vi "Main Window.vi"() -> ()   [LabVIEW 2015]
uses:
  Control Button/Exit.ctl
  Control Button/login.ctl
  Control Button/Logout.ctl
  Control Button/setting.ctl
  Control Button/report.ctl
  Control Button/Manual.ctl
  Control Button/Start.ctl
  Enqueue/Main window Seq/Test selection_1.ctl
  Enqueue/Main window Seq/Test seq_1.ctl
  Galobal variable_TI.vi
  Project Setup/Globle Variable/GR_Servo.vi
panel:
  out "Company Name  2":string
  out "Error":bool
  out "User Name":string
  out "error out":errorcluster
  out "x = y?":bool
  out "Company Name":string
  in  "Sign In":T1
  out "Boolean":bool
  in  "Dashbord":T6
  in  "Login Window":T8 {"User Name" items=["admin", "mmum", "a", "AJAY Kumar", "", "", "", "", "", "", "", "", "", "", "", "", "", "", "", "", "", "", "", "", "", "", "", "", "", "", "", ""]}
  in  "Exit":T9
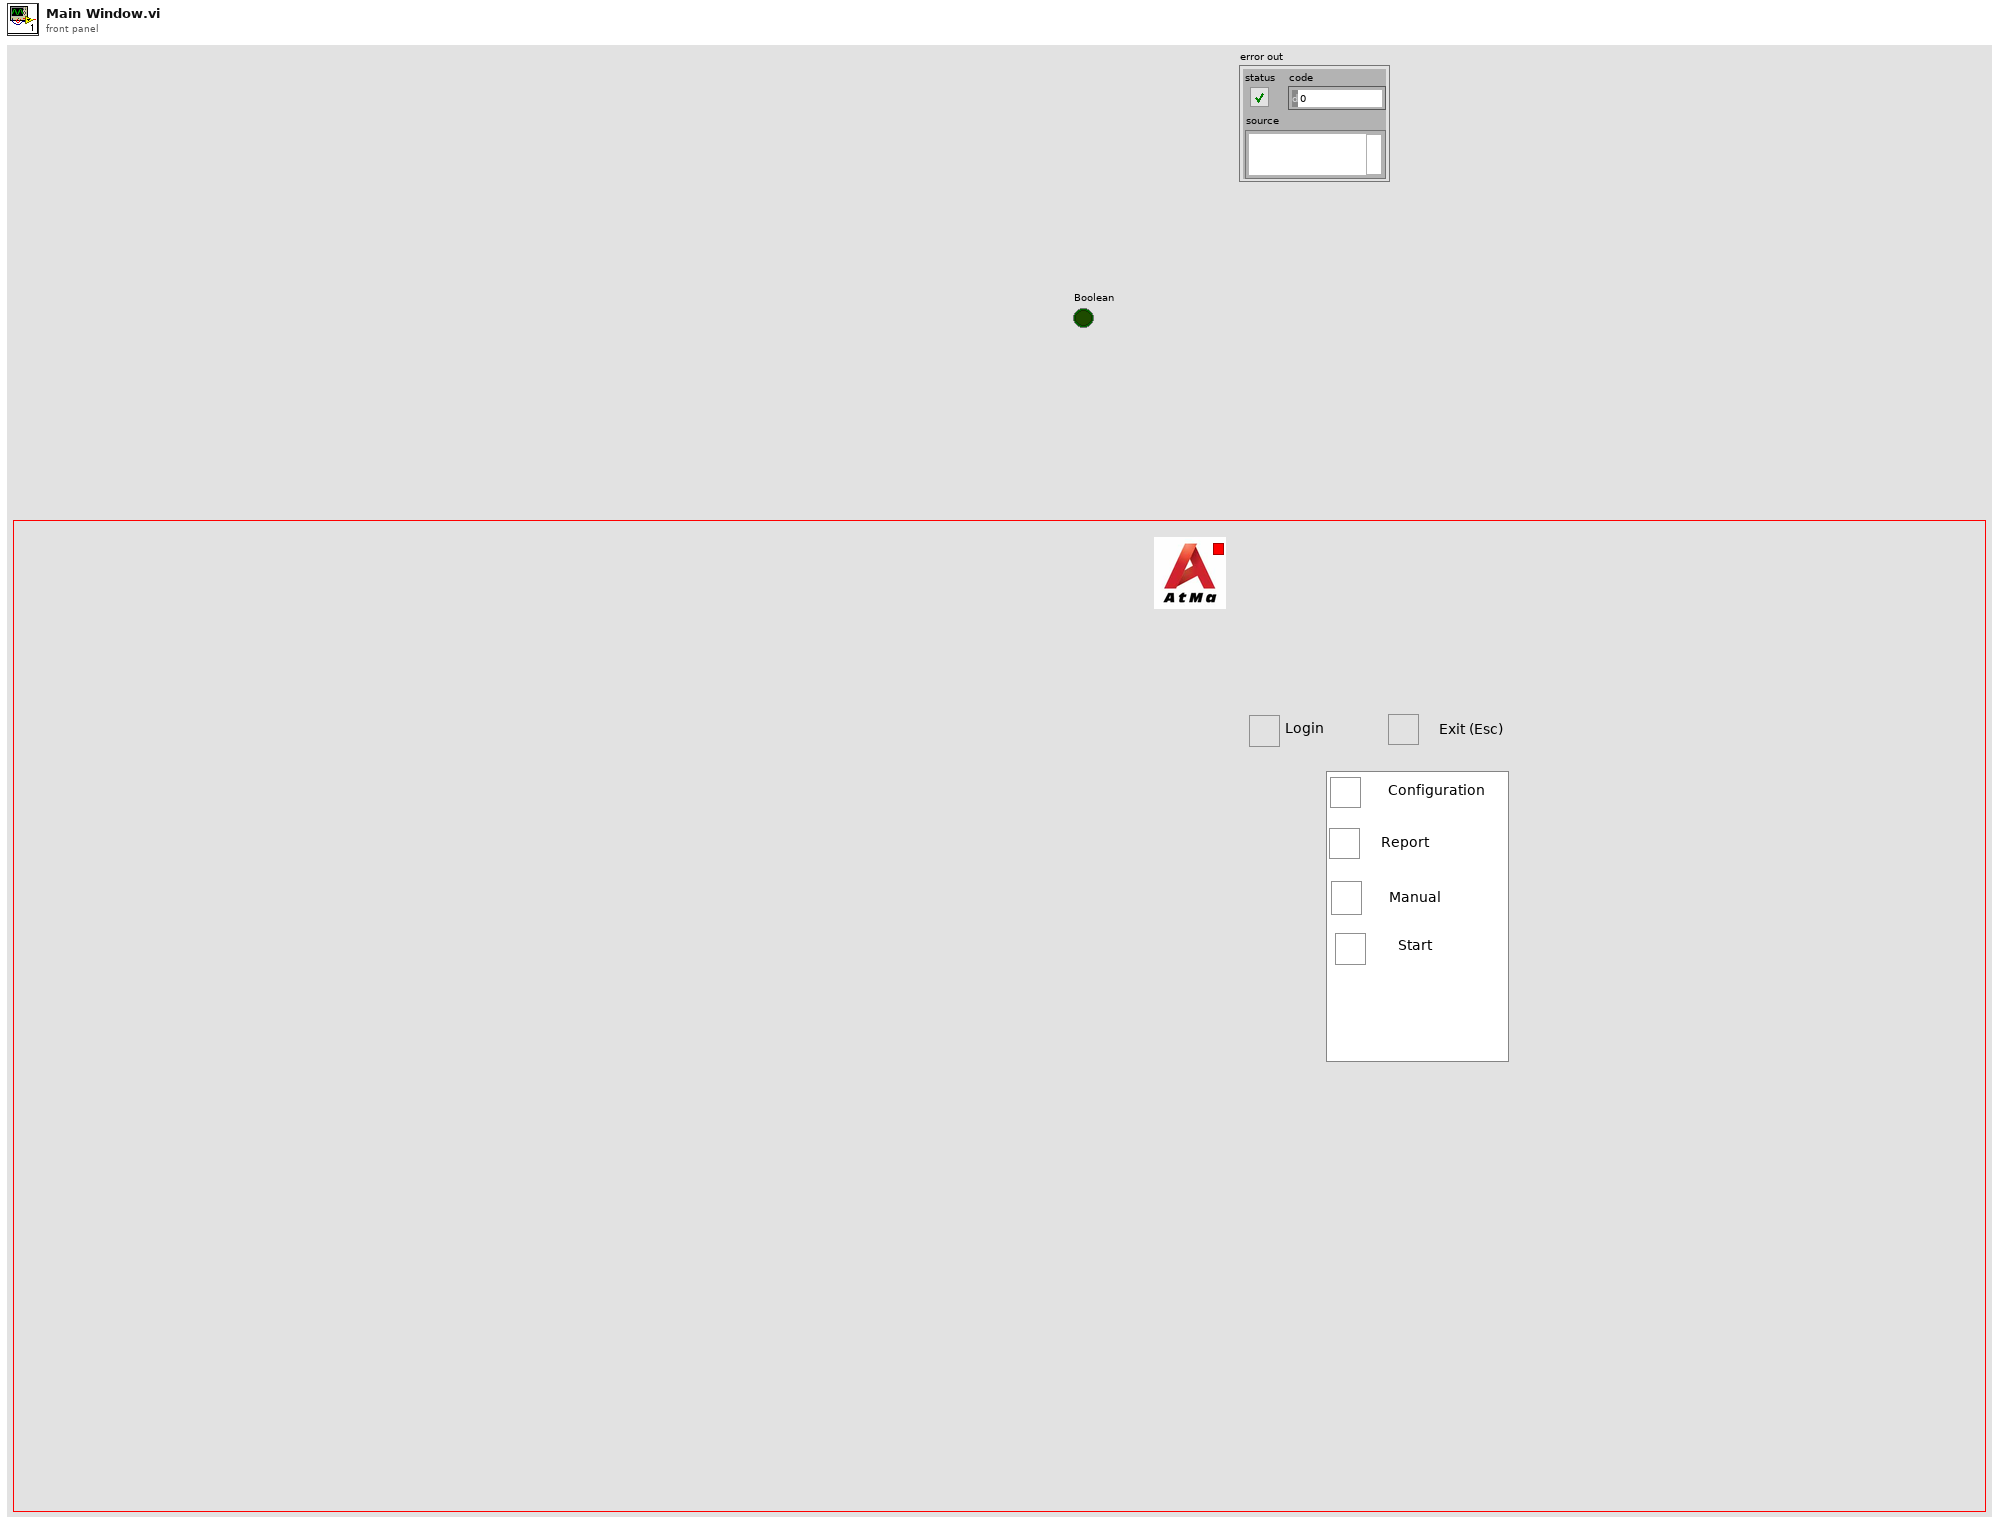
[diagram p1: front panel]
types:
  T1 = typedef "login.ctl" = bool
  T2 = typedef "setting.ctl" = bool
  T3 = typedef "report.ctl" = bool
  T4 = typedef "Manual.ctl" = bool
  T5 = typedef "Start.ctl" = bool
  T6 = cluster{"Setting":T2, "Report":T3, "Manaul":T4, "Start":T5}
  T7 = typedef "Logout.ctl" = bool
  T8 = cluster{"User Name":u16, "Password":string, "Sign In":T1, "Log Out":T7}
  T9 = typedef "Exit.ctl" = bool
  T10 = typedef "Test selection_1.ctl" = enum16{"Init", "Enqueue ", "Enqueue N", "Enqueue in stack", "Enqueue in stack N", "Dequeue", "Dequeue N", "Flush", "Release Queue"}
  T11 = typedef "Test seq_1.ctl" = enum16{"Poll Event", "Login", "Logout", "Confi", "Manual", "Report", "Testing", "Exit"}
  T12 = cluster{"XInput":dbl[], "Y New Value":dbl[], "Avg point":i16}[]
  T13 = cluster{"Slop":dbl[], "Intercept":dbl[], "Average ":i16[]}
  T14 = cluster{"UserName":string[], "Password":string[], "Usertype":string[], "Analog Min":string[], "Analog Max":string[], "DigitalInput Port":string[], "Digital Output Port":string[], "ANalog Port":string[], "IOList":cluster{"DI List_280":string[], "D0List _280":string[], "AI List_280":string[]}}
  T15 = cluster{"DI List_280":string[], "D0List _280":string[], "AI List_280":string[]}
  T16 = cluster{"DigitalInput Port[0]":string, "DigitalInput Port[1]":string, "DigitalInput Port[2]":string, "DigitalInput Port[3]":string, "DigitalInput Port[4]":string, "DigitalInput Port[5]":string, "DigitalInput Port[6]":string, "DigitalInput Port[7]":string, "DigitalInput Port[8]":string, "DigitalInput Port[9]":string, "DigitalInput Port[10]":string, "DigitalInput Port[11]":string, "DigitalInput Port[12]":string, "DigitalInput Port[13]":string, "DigitalInput Port[14]":string, "DigitalInput Port[15]":string, "DigitalInput Port[16]":string, "DigitalInput Port[17]":string, "DigitalInput Port[18]":string, "DigitalInput Port[19]":string, "DigitalInput Port[20]":string}
  T17 = cluster{"Digital Output Port[0]":string, "Digital Output Port[1]":string, "Digital Output Port[2]":string, "Digital Output Port[3]":string, "Digital Output Port[4]":string, "Digital Output Port[5]":string, "Digital Output Port[6]":string, "Digital Output Port[7]":string, "Digital Output Port[8]":string, "Digital Output Port[9]":string, "Digital Output Port[10]":string, "Digital Output Port[11]":string, "Digital Output Port[12]":string, "Digital Output Port[13]":string, "Digital Output Port[14]":string, "Digital Output Port[15]":string, "Digital Output Port[16]":string, "Digital Output Port[17]":string, "Digital Output Port[18]":string, "Digital Output Port[19]":string, "Digital Output Port[20]":string, "Digital Output Port[21]":string, "Digital Output Port[22]":string, "Digital Output Port[23]":string, "Digital Output Port[24]":string, "Digital Output Port[25]":string}
  T18 = cluster{"ANalog Port[0]":string, "ANalog Port[1]":string, "ANalog Port[2]":string, "ANalog Port[3]":string, "ANalog Port[4]":string, "ANalog Port[5]":string, "ANalog Port[6]":string, "ANalog Port[7]":string, "ANalog Port[8]":string, "ANalog Port[9]":string, "ANalog Port[10]":string, "ANalog Port[11]":string, "ANalog Port[12]":string, "ANalog Port[13]":string, "ANalog Port[14]":string, "ANalog Port[15]":string, "ANalog Port[16]":string, "ANalog Port[17]":string, "ANalog Port[18]":string, "ANalog Port[19]":string, "ANalog Port[20]":string, "ANalog Port[21]":string, "ANalog Port[22]":string, "ANalog Port[23]":string, "ANalog Port[24]":string, "ANalog Port[25]":string, "ANalog Port[26]":string, "ANalog Port[27]":string, "ANalog Port[28]":string, "ANalog Port[29]":string, "ANalog Port[30]":string, "ANalog Port[31]":string}
  T19 = enum32{"Invalid", "Standard", "Closed", "Hidden", "Minimized", "Maximized"}
  T20 = enum8{"Enabled", "Disabled", "Disabled and Grayed Out"}
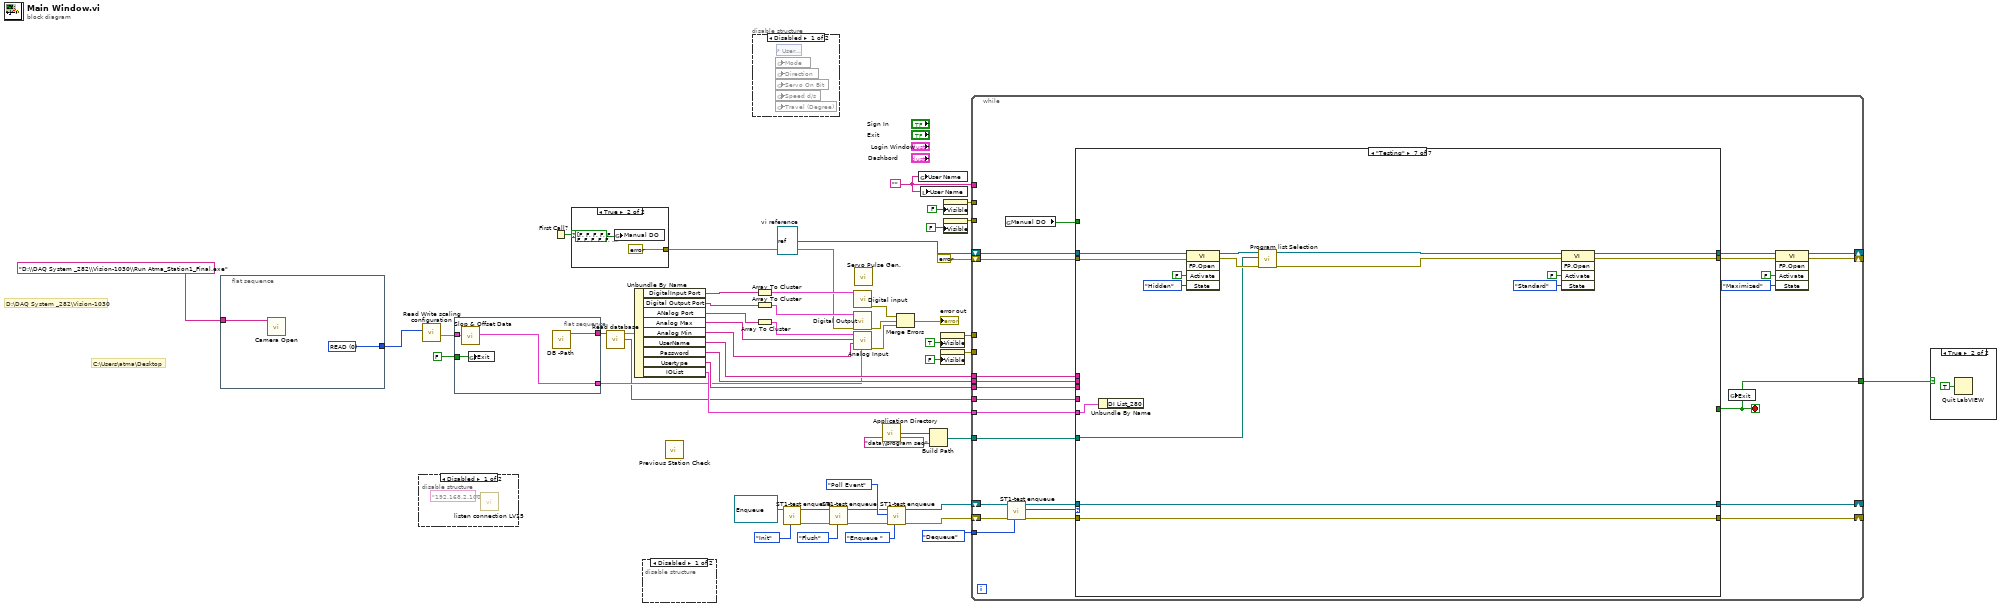
[diagram p0: block diagram]
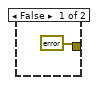
[diagram p5: hidden frame]
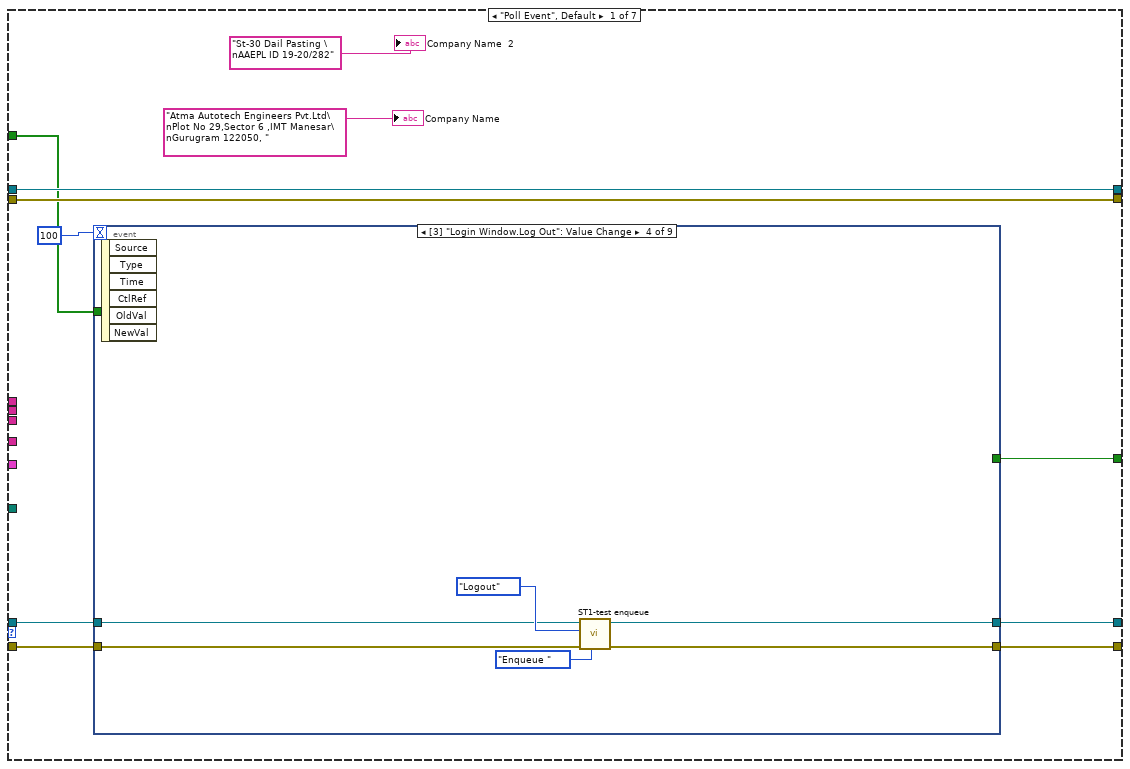
[diagram p7: hidden frame]
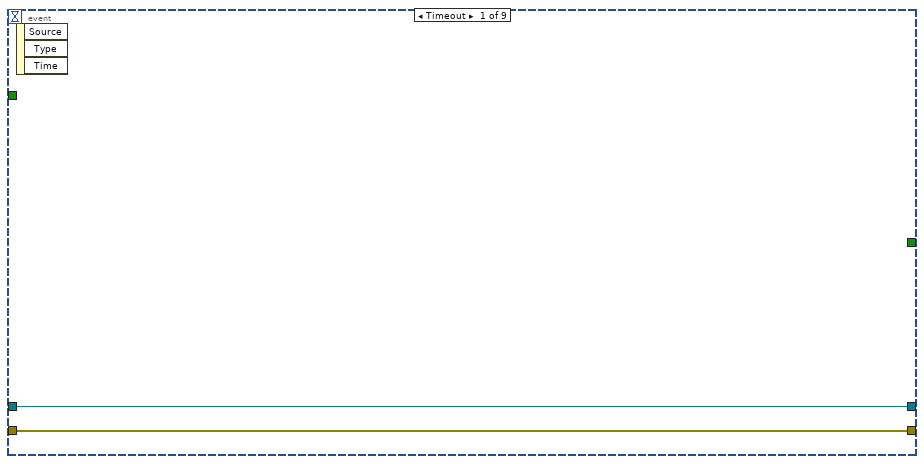
[diagram p8: hidden frame]
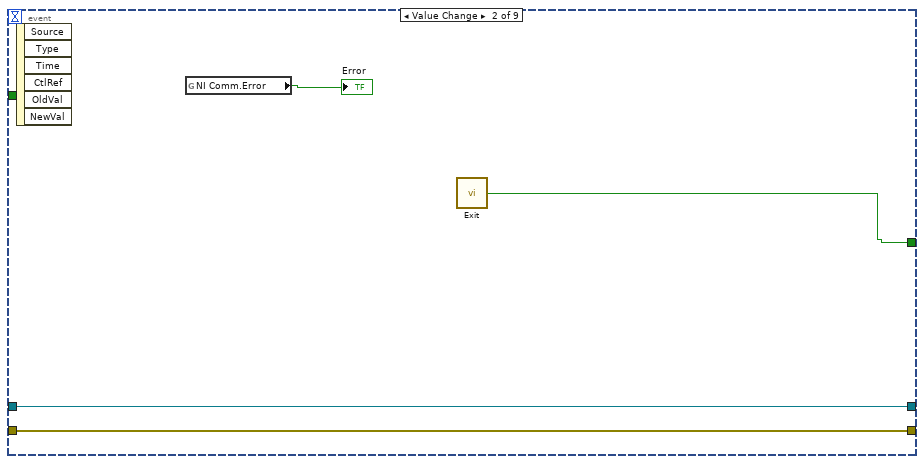
[diagram p9: hidden frame]
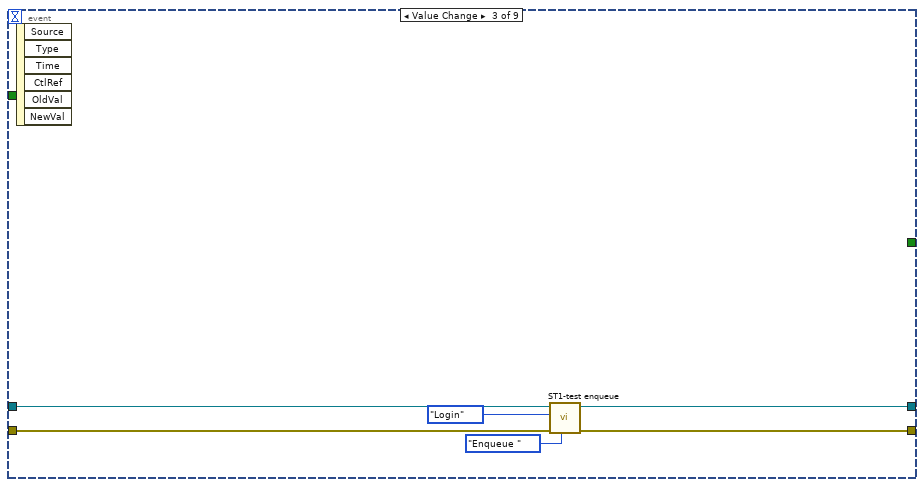
[diagram p10: hidden frame]
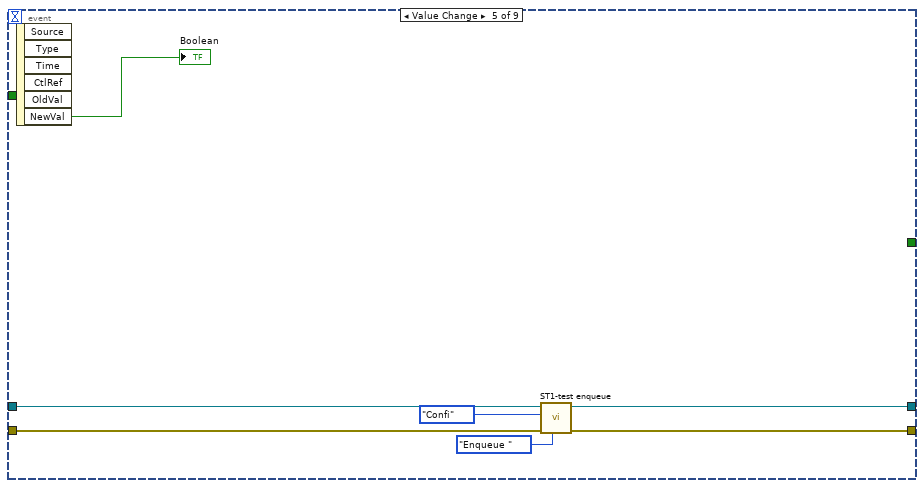
[diagram p11: hidden frame]
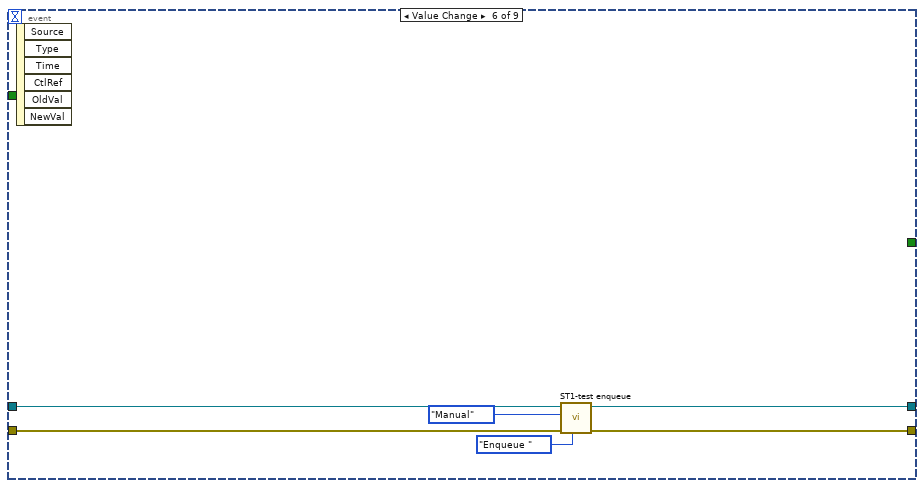
[diagram p12: hidden frame]
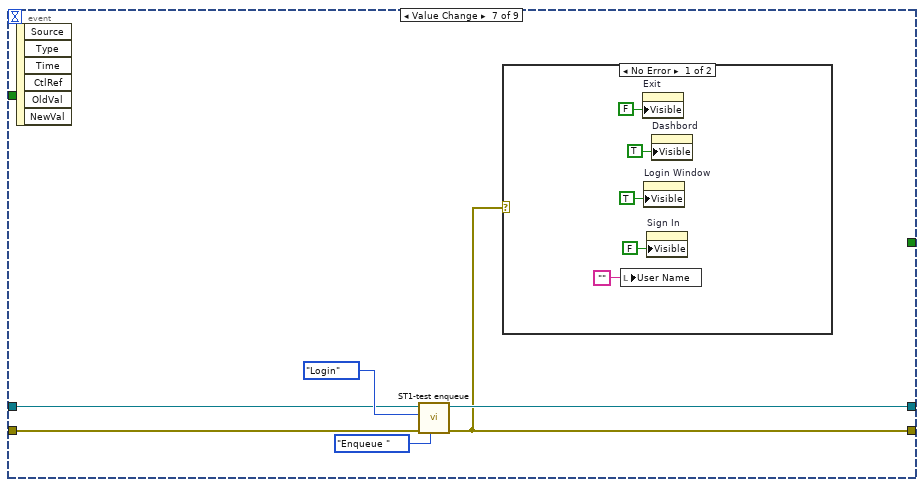
[diagram p13: hidden frame]
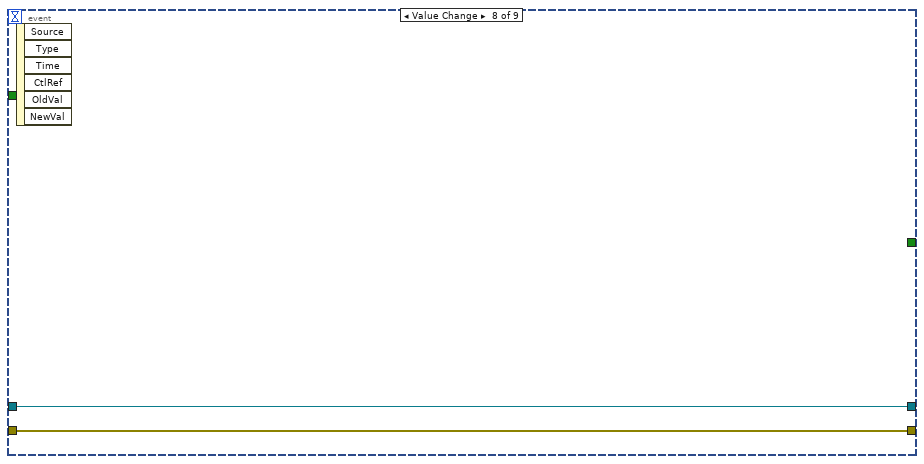
[diagram p15: hidden frame]
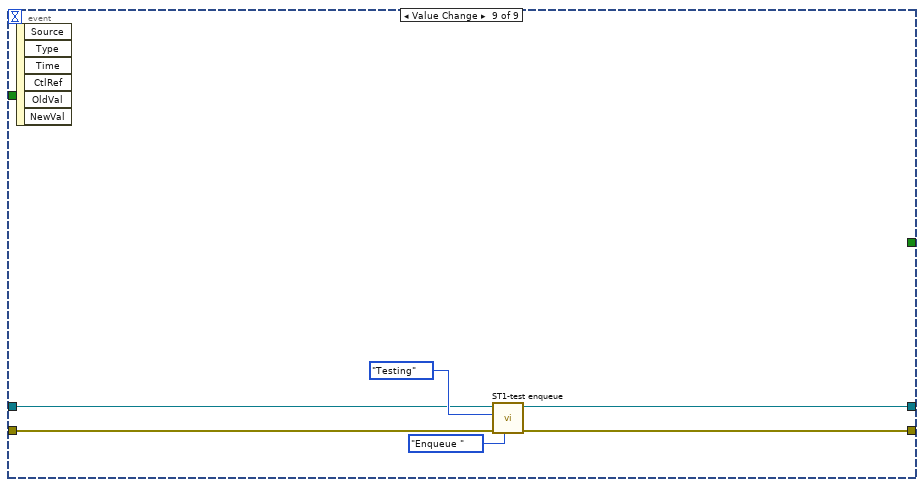
[diagram p16: hidden frame]
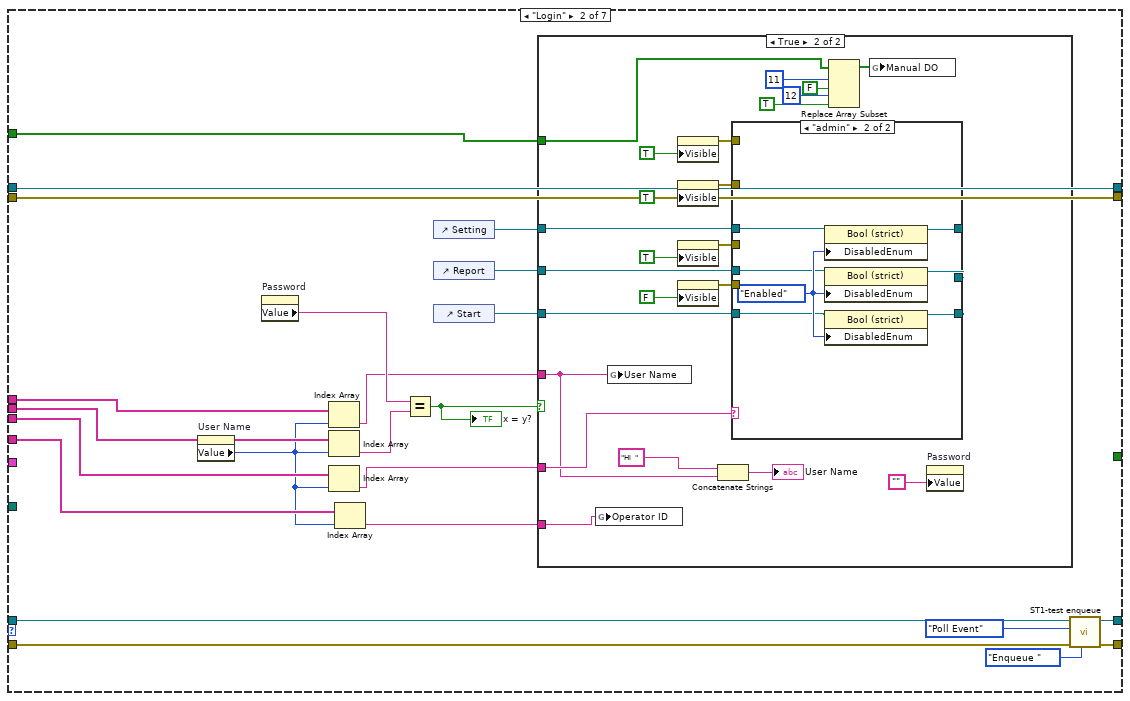
[diagram p17: hidden frame]
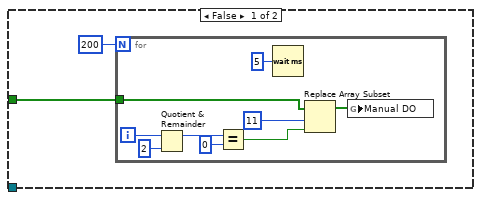
[diagram p18: hidden frame]
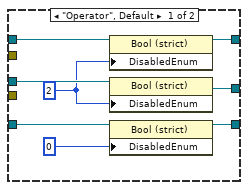
[diagram p19: hidden frame]
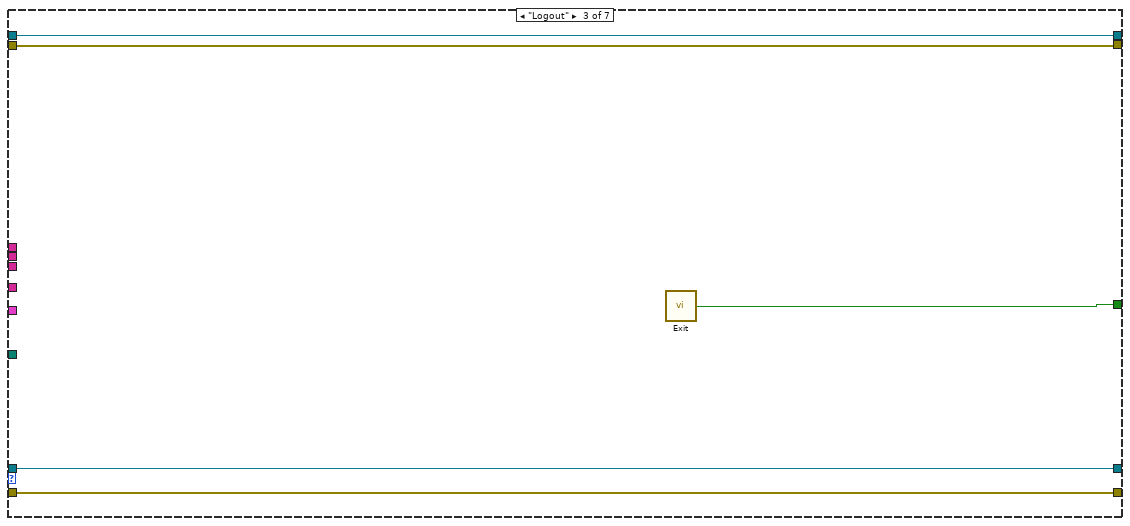
[diagram p20: hidden frame]
diagram:
  w31 = ""
  w41 = refnum<vi> refnum  # vi reference
  w42 = refnum<queue> refnum items=["Poll Event", "Login", "Logout", "Confi", "Manual", "Report", "Testing", "Exit"] ("queue in")
  # "D:\\DAQ System _282\\Vision-1030"
  # "C:\\Users\\atma\\Desktop"
  n1 = flat-sequence {
    tunnel: "D:\\DAQ System _282\\Vision-1030\\Run Atma_Station1_Final.exe" ("command line") -> [w55]
    tunnel: [w54] -> w3
    frame #0 {
      w54 = u16 0 items=["READ", "WRITE"] ("Read/Write")
      n2 = call "Camera Open.vi"("command line"=w55) -> ()  [unwired: 11 in]
    }
  }
  n3 = disable-structure shown="Disabled" {
    frame Disabled {
      n4 = call "listen connection LV15.vi"("service name"="192.168.2.100") -> ()  [unwired: 8 in, 2 out]
    }
    frame Enabled {
    }
  }
  n5 = call "Read Write scaling configuration.vi"("Read/Write"=w3) -> ("Output"=w16:T12)  [unwired: 4 in, 2 out]
  n6 = flat-sequence {
    tunnel: [w60] -> w30
    tunnel: w16 -> [w59]
    tunnel: [w58] -> w15
    tunnel: FALSE ("Exit") -> [w57]
    frame #0 {
      n7 = call "Slop & Offset Data.vi"("Input"=w59) -> ("Cluster"=w58:T13)  [unwired: 10 in]
      n8 = global write "Galobal variable_TI.vi" "Exit"(w57) -> ()
      n9 = call "DB -Path.vi"() -> ("String"=w60:string)  [unwired: 11 in]
    }
  }
  n10 = First Call?() -> (First Call?: T/F=w6:bool)
  n11 = case shown="True" w6 {
    tunnel: [errorcluster {"status"=FALSE, "code"=0, "source"=""} ("error constant") errorcluster {"status"=FALSE, "code"=0, "source"=""} ("error constant")] -> w5
    frame False {
    }
    frame True {
      n12 = global write "Galobal variable_TI.vi" "Manual DO"(bool[] [FALSE, FALSE, FALSE, FALSE, FALSE, FALSE, FALSE, FALSE, FALSE, FALSE, FALSE, FALSE, FALSE, FALSE, FALSE, FALSE, FALSE, FALSE, FALSE, FALSE, FALSE, FALSE, FALSE, FALSE, FALSE, FALSE, FALSE, FALSE, FALSE, FALSE] ("Manual DO")) -> ()
    }
  }
  n13 = call "Read database.vi"("String"=w30) -> ("Operator ID"=w1:string[], "DB Data"=w29:T14)  [unwired: 2 in, 1 out]
  n14 = Unbundle By Name(w29) -> ("DigitalInput Port"=w28:string[], "Digital Output Port"=w26:string[], "ANalog Port"=w24:string[], "Analog Max"=w22:string[], "Analog Min"=w21:string[], "UserName"=w20:string[], "Password"=w19:string[], "Usertype"=w18:string[], "IOList"=w17:T15)
  n15 = disable-structure shown="Disabled" {
    frame Disabled {
    }
    frame Enabled {
    }
  }
  n16 = call "Previous Station Check.vi"() -> ()  [unwired: 12 in]
  n17 = disable-structure shown="Disabled" {
    frame Disabled {
      n18 = global read "GR_Servo.vi" "Mode"() -> ()  [unwired: 1 in]
      n19 = global read "GR_Servo.vi" "Direction"() -> ()  [unwired: 1 in]
      n20 = global read "GR_Servo.vi" "Servo On Bit"() -> ()  [unwired: 1 in]
      n21 = global read "GR_Servo.vi" "Speed d/s"() -> ()  [unwired: 1 in]
      n22 = global read "GR_Servo.vi" "Travel (Degree)"() -> ()  [unwired: 1 in]
      n23 = control-ref of="User Name"() -> ()  [unwired: 1 out]
    }
    frame Enabled {
    }
  }
  n24 = Array To Cluster(array=w28) -> (cluster=w27:T16)
  n25 = Array To Cluster(array=w26) -> (cluster=w25:T17)
  n26 = Array To Cluster(array=w24) -> (cluster=w23:T18)
  n27 = call "ST1-test enqueue.vi"("Enum Selection"=Test_selection_1."Init", "queue in"=w42) -> ("error out"=w51:errorcluster, "queue Out"=w47:refnum<queue>)  [unwired: 6 in, 1 out]
  n28 = call "ST1-test enqueue.vi"("Enum Selection"=Test_selection_1."Flush", "Error In"=w51, "queue in"=w47) -> ("error out"=w49:errorcluster, "queue Out"=w46:refnum<queue>)  [unwired: 5 in, 1 out]
  n29 = call "Digital Output.vi"("error in"=w5, "DAQmx OutPut Setting"=w25) -> ("error out"=w13:errorcluster)  [unwired: 8 in, 1 out]
  n30 = call "Digital input.vi"("DAQmx InPut Setting"=w27) -> ("error out"=w11:errorcluster)  [unwired: 9 in, 1 out]
  n31 = call "Analog Input.vi"("clai. Parmeter"=w15, "Min Value"=w21, "Max Value"=w22, "DAQmx Analog Input Setting"=w23) -> ("error out"=w12:errorcluster)  [unwired: 6 in, 1 out]
  n32 = call "Servo Pulse Gen..vi"() -> ()  [unwired: 12 in]
  n33 = call <vilib>:"Application Directory.vi"() -> ("Application Directory"=w9:path)
  n34 = call "ST1-test enqueue.vi"("Enum Selection"=Test_selection_1."Enqueue ", "Error In"=w49, "Enqueue"=Test_seq_1."Poll Event", "queue in"=w46) -> ("error out"=w44:errorcluster, "queue Out"=w45:refnum<queue>)  [unwired: 4 in, 1 out]
  n35 = Merge Errors(w11, w13, w12) -> (→"error out":errorcluster)
  n36 = global write "Galobal variable_TI.vi" "User Name"(w31) -> ()
  n37 = local write "User Name"(w31) -> ()
  n38 = Build Path(base path=w9, name or relative path="data\\program seq") -> (appended path=w7:path)
  n39 = property on="Login Window" class="Clust (strict)"("Visible"=TRUE) -> (error out=w36:errorcluster)  [unwired: 2 in, 1 out]
  n40 = property on="Sign In" class="Bool (strict)"("Visible"=FALSE) -> (error out=w35:errorcluster)  [unwired: 2 in, 1 out]
  n41 = property on="Exit" class="Bool (strict)"("Visible"=FALSE) -> (error out=w33:errorcluster)  [unwired: 2 in, 1 out]
  n42 = property on="Dashbord" class="Clust (strict)"("Visible"=FALSE) -> (error out=w38:errorcluster)  [unwired: 2 in, 1 out]
  n43 = while {
    shift-right: [w81] -> _
    shift-left: w45 -> [w87]
    shift-right: [w80] -> _
    shift-left: w44 -> [w86]
    tunnel: Test_selection_1."Dequeue" ("Enum Selection") -> [w85]
    shift-right: [w72] -> _
    shift-left: errorcluster {"status"=FALSE, "code"=0, "source"=""} ("error out") -> [w78]
    shift-right: [w73] -> _
    shift-left: w41 -> [w79]
    tunnel: w38 -> [_]
    tunnel: w36 -> [_]
    tunnel: w35 -> [_]
    tunnel: w33 -> [_]
    tunnel: w31 -> [_]
    tunnel: w20 -> [w71]
    tunnel: w19 -> [w70]
    tunnel: w18 -> [w69]
    tunnel: w17 -> [w68]
    tunnel: w7 -> [w67]
    tunnel: [w65] -> w4
    tunnel: w1 -> [w64]
    stop <- w65 stop-if-true
    n44 = global read "Galobal variable_TI.vi" "Manual DO"() -> (w66:bool[])
    n45 = call "ST1-test enqueue.vi"("Enum Selection"=w85, "Error In"=w86, "queue in"=w87) -> ("error out"=w82:errorcluster, "D-enqueue"=w84:T11, "queue Out"=w83:refnum<queue>)  [unwired: 5 in]
    n46 = case shown="\"Testing\"" w84 {
      tunnel: [w96 _ w221 _ _ _ _] -> w65
      tunnel: w83 -> [w97 w153 w225 w239 w247 w256 w272]
      tunnel: w82 -> [w98 w152 w224 w238 w246 w255 w271]
      tunnel: [w95 w156 w225 w239 w247 w256 w272] -> w81
      tunnel: [w94 w155 w224 w238 w246 w255 w271] -> w80
      tunnel: [w93 w165 w223 w233 w242 w254 w259] -> w75
      tunnel: [w92 w164 w222 w232 w243 w253 w257] -> w74
      tunnel: w79 -> [w93 w165 w223 w231 w244 w254 w264]
      tunnel: w78 -> [w92 w164 w222 w230 w245 w253 w267]
      tunnel: w71 -> [_ w162 _ _ _ _ _]
      tunnel: w70 -> [_ w161 _ _ _ _ _]
      tunnel: w69 -> [_ w160 _ _ _ _ _]
      tunnel: w68 -> [_ _ _ w226 w241 _ w270]
      tunnel: w67 -> [_ _ _ _ _ _ w263]
      tunnel: w66 -> [w89 w154 _ _ _ _ _]
      tunnel: w64 -> [_ w151 _ _ _ _ _]
      frame "Poll Event", Default {
        n47 = event shown="[3] \"Login Window.Log Out\": Value Change" {
          selector: _ -> [_ _ _ _ _ _ _ _ _]
          dyn-events: _ -> [_ _ _ _ _ _ _ _ _]
          timeout: 100 -> [_ _ _ _ _ _ _ _ _]
          tunnel: [_ w102 _ _ _ _ _ _ _] -> w96
          tunnel: w98 -> [w99 w103 w108 w111 w119 w127 w133 w141 w145]
          tunnel: w97 -> [w100 w104 w109 w112 w120 w125 w132 w142 w146]
          tunnel: [w100 w104 w107 w114 w118 w124 w131 w142 w144] -> w95
          tunnel: [w99 w103 w106 w113 w117 w126 w130 w141 w143] -> w94
          tunnel: w89 -> [_ _ _ _ _ _ _ _ _]
          event Timeout {
            n48 = event-data() -> ()  [unwired: 1 in, 3 out]
          }
          event Value Change {
            n49 = event-data() -> ()  [unwired: 1 in, 6 out]
            n50 = global read "Galobal variable_TI.vi" "NI Comm.Error"() -> (→"Error":bool)
            n51 = call "Exit.vi"() -> ("Exit"=w102:bool)  [unwired: 1 in]
          }
          event Value Change {
            n52 = event-data() -> ()  [unwired: 1 in, 6 out]
            n53 = call "ST1-test enqueue.vi"("Enum Selection"=Test_selection_1."Enqueue ", "Error In"=w108, "Enqueue"=Test_seq_1."Login", "queue in"=w109) -> ("error out"=w106:errorcluster, "queue Out"=w107:refnum<queue>)  [unwired: 4 in, 1 out]
          }
          event Value Change {
            n54 = event-data() -> ()  [unwired: 1 in, 6 out]
            n55 = call "ST1-test enqueue.vi"("Enum Selection"=Test_selection_1."Enqueue ", "Error In"=w111, "Enqueue"=Test_seq_1."Logout", "queue in"=w112) -> ("error out"=w113:errorcluster, "queue Out"=w114:refnum<queue>)  [unwired: 4 in, 1 out]
          }
          event Value Change {
            n56 = event-data() -> ("NewVal"=→"Boolean":T2)  [unwired: 1 in, 5 out]
            n57 = call "ST1-test enqueue.vi"("Enum Selection"=Test_selection_1."Enqueue ", "Error In"=w119, "Enqueue"=Test_seq_1."Confi", "queue in"=w120) -> ("error out"=w117:errorcluster, "queue Out"=w118:refnum<queue>)  [unwired: 4 in, 1 out]
          }
          event Value Change {
            n58 = event-data() -> ()  [unwired: 1 in, 6 out]
            n59 = call "ST1-test enqueue.vi"("Enum Selection"=Test_selection_1."Enqueue ", "Error In"=w127, "Enqueue"=Test_seq_1."Manual", "queue in"=w125) -> ("error out"=w126:errorcluster, "queue Out"=w124:refnum<queue>)  [unwired: 4 in, 1 out]
          }
          event Value Change {
            n60 = event-data() -> ()  [unwired: 1 in, 6 out]
            n61 = call "ST1-test enqueue.vi"("Enum Selection"=Test_selection_1."Enqueue ", "Error In"=w133, "Enqueue"=Test_seq_1."Login", "queue in"=w132) -> ("error out"=w130:errorcluster, "queue Out"=w131:refnum<queue>)  [unwired: 4 in, 1 out]
            n62 = case shown="No Error" w130 {
              frame No Error {
                n63 = local write "User Name"("") -> ()
                n64 = property on="Exit" class="Bool (strict)"("Visible"=FALSE) -> ()  [unwired: 2 in, 2 out]
                n65 = property on="Login Window" class="Clust (strict)"("Visible"=TRUE) -> ()  [unwired: 2 in, 2 out]
                n66 = property on="Sign In" class="Bool (strict)"("Visible"=FALSE) -> ()  [unwired: 2 in, 2 out]
                n67 = property on="Dashbord" class="Clust (strict)"("Visible"=TRUE) -> ()  [unwired: 2 in, 2 out]
              }
              frame Error {
              }
            }
          }
          event Value Change {
            n68 = event-data() -> ()  [unwired: 1 in, 6 out]
          }
          event Value Change {
            n69 = event-data() -> ()  [unwired: 1 in, 6 out]
            n70 = call "ST1-test enqueue.vi"("Enum Selection"=Test_selection_1."Enqueue ", "Error In"=w145, "Enqueue"=Test_seq_1."Testing", "queue in"=w146) -> ("error out"=w143:errorcluster, "queue Out"=w144:refnum<queue>)  [unwired: 4 in, 1 out]
          }
        }
        "Company Name" <- "Atma Autotech Engineers Pvt.Ltd\nPlot No 29,Sector 6 ,IMT Manesar\nGurugram 122050, " ("string")
        "Company Name  2" <- "St-30 Dail Pasting \nAAEPL ID 19-20/282" ("string")
      }
      frame "Login" {
        n71 = property on="User Name" class="Ring (strict)"() -> ("Value"=w150:u16)  [unwired: 2 in, 2 out]
        n72 = property on="Password" class="Str"() -> ("Value"=w170:string)  [unwired: 2 in, 2 out]
        n73 = Index Array(array=w162, index=w150) -> (element=w163:string)
        n74 = Index Array(array=w161, index=w150) -> (element=w171:string)
        n75 = Index Array(array=w160, index=w150) -> (element=w169:string)
        n76 = Index Array(array=w151, index=w150) -> (element=w149:string)
        n77 = Equal?(x=w170, y=w171) -> (x = y?=w159:bool)
        "x = y?" <- w159
        n78 = control-ref of="Setting"() -> (w168:refnum<vi>)
        n79 = control-ref of="Report"() -> (w166:refnum<vi>)
        n80 = control-ref of="Start"() -> (w167:refnum<vi>)
        n81 = case shown="True" w159 {
          tunnel: w169 -> [_ w201]
          tunnel: w168 -> [_ w205]
          tunnel: w166 -> [_ w204]
          tunnel: w167 -> [_ w203]
          tunnel: w163 -> [_ w184]
          tunnel: w154 -> [w172 w188]
          tunnel: w149 -> [_ w183]
          frame False {
            n82 = for {
              N: 200 -> [_]
              tunnel: w172 -> [w174]
              i -> [w182]
              n83 = Quotient & Remainder(x=w182, y=2) -> (x-y*floor(x/y)=w180:i32)  [unwired: 1 out]
              n84 = Equal?(x=w180, y=0) -> (x = y?=w177:bool)
              n85 = Wait (ms)(milliseconds to wait=u32 5) -> ()  [unwired: 1 out]
              n86 = Replace Array Subset(array=w174, new element=w177, index=11) -> (w175:bool[])
              n87 = global write "Galobal variable_TI.vi" "Manual DO"(w175) -> ()
            }
          }
          frame True {
            n88 = global write "Galobal variable_TI.vi" "Operator ID"(w183) -> ()
            n89 = global write "Galobal variable_TI.vi" "User Name"(w184) -> ()
            n90 = property on="Exit" class="Bool (strict)"("Visible"=TRUE) -> (error out=w192:errorcluster)  [unwired: 2 in, 1 out]
            n91 = property on="Dashbord" class="Clust (strict)"("Visible"=TRUE) -> (error out=w197:errorcluster)  [unwired: 2 in, 1 out]
            n92 = property on="Sign In" class="Bool (strict)"("Visible"=TRUE) -> (error out=w196:errorcluster)  [unwired: 2 in, 1 out]
            n93 = property on="Login Window" class="Clust (strict)"("Visible"=FALSE) -> (error out=w198:errorcluster)  [unwired: 2 in, 1 out]
            n94 = Concatenate Strings("Hi  " ("string"), w184) -> (→"User Name":string)
            n95 = case shown="\"admin\"" w201 {
              tunnel: [w213 w219] -> _
              tunnel: [w212 w218] -> _
              tunnel: [w211 w217] -> _
              tunnel: w205 -> [w210 w216]
              tunnel: w204 -> [w209 w215]
              tunnel: w203 -> [w208 w214]
              tunnel: w198 -> [_ _]
              tunnel: w197 -> [_ _]
              tunnel: w196 -> [_ _]
              tunnel: w192 -> [_ _]
              frame "Operator", Default {
                w206 = 2
                n96 = property class="Bool (strict)"(reference=w210, "DisabledEnum"=w206) -> (reference out=w213:refnum<vi>)  [unwired: 1 in, 1 out]
                n97 = property class="Bool (strict)"(reference=w209, "DisabledEnum"=w206) -> (reference out=w212:refnum<vi>)  [unwired: 1 in, 1 out]
                n98 = property class="Bool (strict)"(reference=w208, "DisabledEnum"=0) -> (reference out=w211:refnum<vi>)  [unwired: 1 in, 1 out]
              }
              frame "admin" {
                w220 = T20."Enabled" ("Disabled")
                n99 = property class="Bool (strict)"(reference=w216, "DisabledEnum"=w220) -> (reference out=w219:refnum<vi>)  [unwired: 1 in, 1 out]
                n100 = property class="Bool (strict)"(reference=w215, "DisabledEnum"=w220) -> (reference out=w218:refnum<vi>)  [unwired: 1 in, 1 out]
                n101 = property class="Bool (strict)"(reference=w214, "DisabledEnum"=w220) -> (reference out=w217:refnum<vi>)  [unwired: 1 in, 1 out]
              }
            }
            n102 = Replace Array Subset(array=w188, new element #1=FALSE ("new element/subarray"), index #1=11 ("index"), new element #2=TRUE ("new element/subarray"), index #2=12 ("index")) -> (w189:bool[])
            n103 = global write "Galobal variable_TI.vi" "Manual DO"(w189) -> ()
            n104 = property on="Password" class="Str"("Value"="") -> ()  [unwired: 2 in, 2 out]
          }
        }
        n105 = call "ST1-test enqueue.vi"("Enum Selection"=Test_selection_1."Enqueue ", "Error In"=w152, "Enqueue"=Test_seq_1."Poll Event", "queue in"=w153) -> ("error out"=w155:errorcluster, "queue Out"=w156:refnum<queue>)  [unwired: 4 in, 1 out]
      }
      frame "Logout" {
        n106 = call "Exit.vi"() -> ("Exit"=w221:bool)  [unwired: 1 in]
      }
      frame "Confi" {
        n107 = invoke class="VI" method="FP.Open"(reference=w231, error in=w230, "Activate"=FALSE ("Activate?"), "State"=T19."Hidden") -> (reference out=w227:refnum<vi>, error out=w229:errorcluster)  [unwired: 1 in, 3 out]
        n108 = call "General Config.vi"("error In"=w229, "IOList"=w226) -> ("error out"=w228:errorcluster)  [unwired: 8 in, 1 out]
        n109 = invoke class="VI" method="FP.Open"(reference=w227, error in=w228, "Activate"=FALSE ("Activate?"), "State"=T19."Standard") -> (reference out=w233:refnum<vi>, error out=w232:errorcluster)  [unwired: 1 in, 3 out]
      }
      frame "Manual" {
        w240 = TRUE ("Manual CMD")
        n110 = global write "Galobal variable_TI.vi" "Manual CMD"(w240) -> ()
        n111 = flat-sequence {
          tunnel: w245 -> [w252]
          tunnel: w244 -> [w251]
          tunnel: [w250] -> w243
          tunnel: [w249] -> w242
          tunnel: w241 -> [w248]
          tunnel: w240 -> [_]
          frame #0 {
            n112 = call "Manual.vi"("vi reference"=w251, "error in (no error)"=w252, "IOList_280"=w248) -> ("error out"=w250:errorcluster, "Out reference"=w249:refnum<vi>)  [unwired: 7 in]
          }
        }
      }
      frame "Report" {
      }
      frame "Testing" {
        n113 = Unbundle By Name(w270) -> ()  [unwired: 1 out]
        n114 = invoke class="VI" method="FP.Open"(reference=w264, error in=w267, "Activate"=FALSE ("Activate?"), "State"=T19."Hidden") -> (reference out=w266:refnum<vi>, error out=w265:errorcluster)  [unwired: 1 in, 3 out]
        n115 = call "Program list Selection.vi"("error in"=w265, "Filepath"=w263, "vi referenceIn"=w266) -> ("error out"=w258:errorcluster, "vi reference Out"=w260:refnum<vi>)  [unwired: 5 in, 2 out]
        n116 = invoke class="VI" method="FP.Open"(reference=w260, error in=w258, "Activate"=FALSE ("Activate?"), "State"=T19."Standard") -> (reference out=w259:refnum<vi>, error out=w257:errorcluster)  [unwired: 1 in, 3 out]
      }
    }
    n117 = global write "Galobal variable_TI.vi" "Exit"(w65) -> ()
    n118 = invoke class="VI" method="FP.Open"(reference=w75, error in=w74, "Activate"=FALSE ("Activate?"), "State"=T19."Maximized") -> (reference out=w73:refnum<vi>, error out=w72:errorcluster)  [unwired: 1 in, 3 out]
  }
  n119 = case shown="True" w4 {
    frame False {
    }
    frame True {
      n120 = Quit LabVIEW(quit? (T)=TRUE) -> ()
    }
  }
